vi "IZRCSM_Check_chosen_field (SubVI).vi"(8 "Error In":errorcluster, 11 "Settings in":T2) -> (0 "Error Out":errorcluster, 3 "Settings out":T2)   [LabVIEW 2018]
uses:
  IZRCSM.ctl
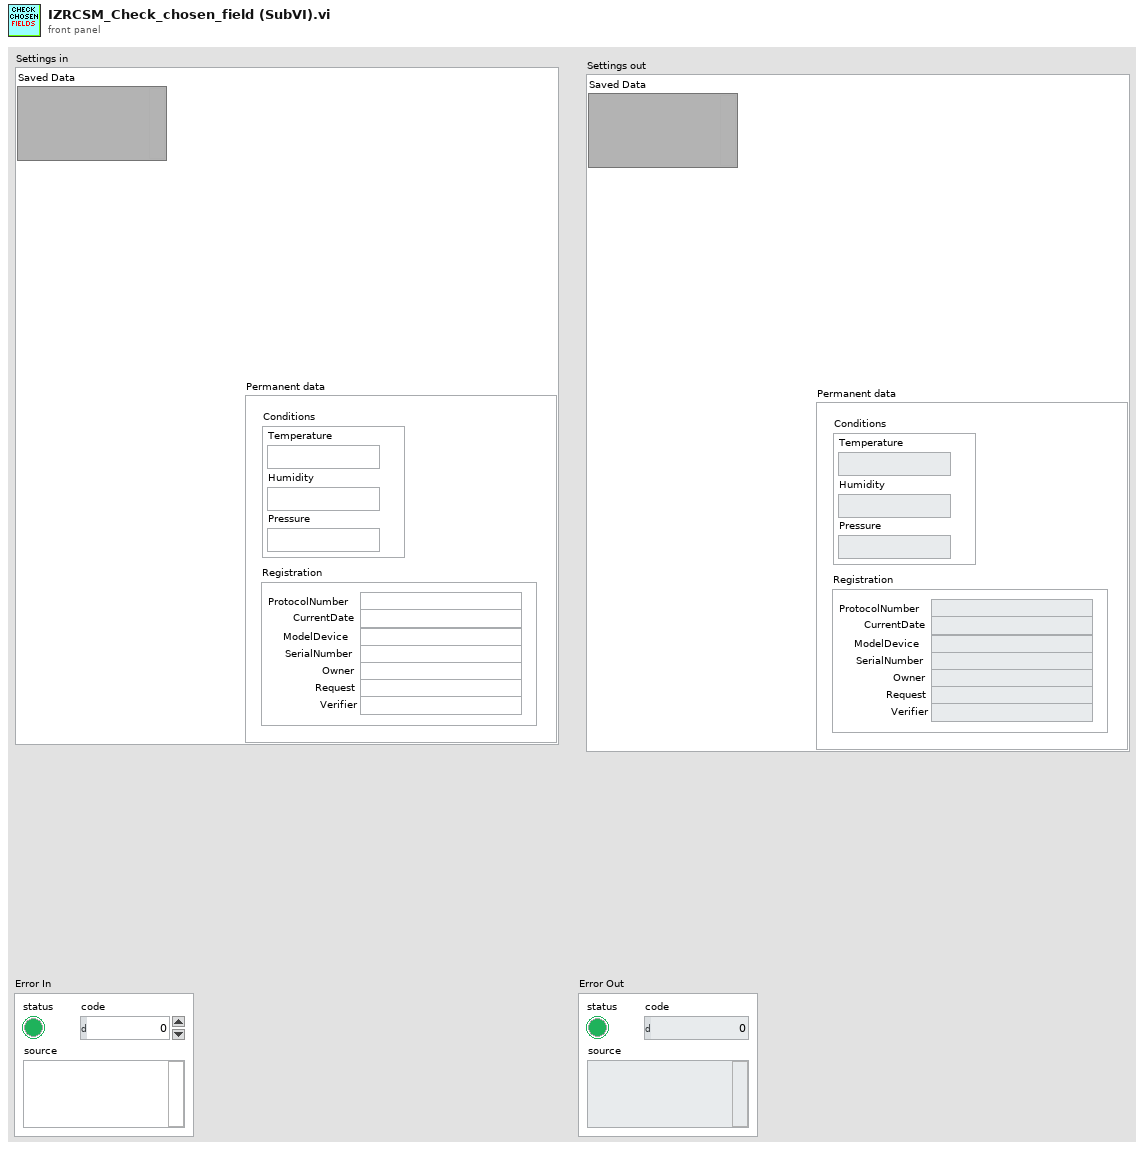
[diagram p1: front panel]
types:
  T1 = typedef "IZRCSM.ctl" = cluster{"Conditions":cluster{"Temperature":string, "Humidity":string, "Pressure":string}, "Registration":cluster{"ProtocolNumber":string, "CurrentDate":string, "ModelDevice":string, "SerialNumber":string, "Owner":string, "Request":string, "Verifier":string}}
  T2 = cluster{"Saved Data":variant, "Permanent data":T1}
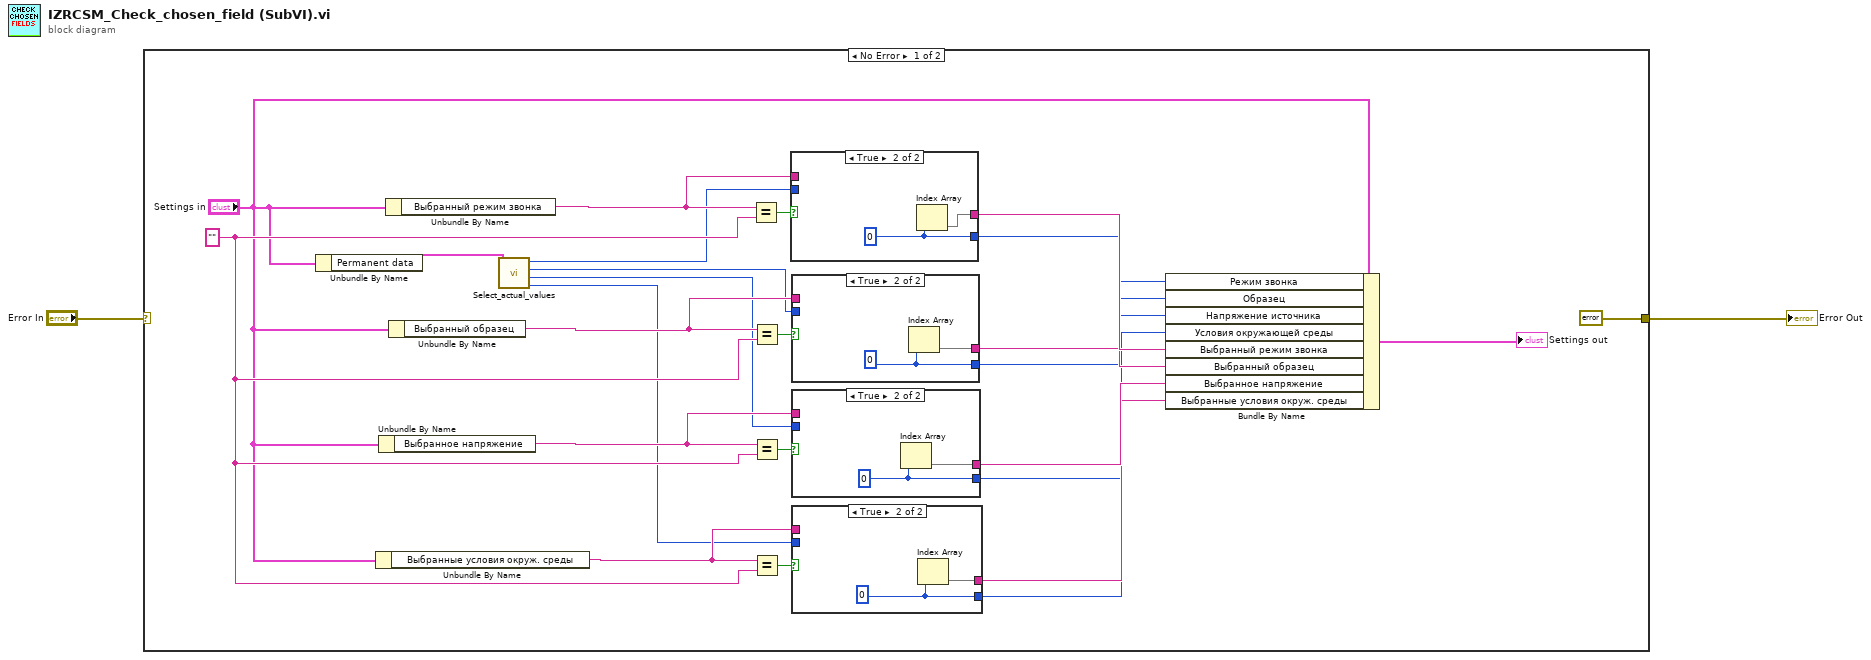
[diagram p0: block diagram]
diagram:
  n1 = case shown="No Error" "Error In" {
    selector: "Error In" -> [_ w48]
    tunnel: [errorcluster {"status"=FALSE, "code"=0, "source"=""} ("error IO") w48] -> w1
    frame No Error {
      w19 = "" ("replace string (\"\")")
      n2 = Unbundle By Name("Settings in") -> ("Permanent data"=w7:T1)
      n3 = Unbundle By Name("Settings in") -> ("Выбранные условия окруж. среды"=w21:string)
      n4 = Unbundle By Name("Settings in") -> ("Выбранное напряжение"=w22:string)
      n5 = Unbundle By Name("Settings in") -> ("Выбранный режим звонка"=w23:string)
      n6 = Unbundle By Name("Settings in") -> ("Выбранный образец"=w24:string)
      n7 = call "Select_actual_values.vi"("CSMinfo in"=w7) -> ("Условия окружающей среды"=w3:u16, "Напряжение источника"=w4:u16, "Образец"=w5:u16, "Режим звонка"=w6:u16)  [unwired: 7 in]
      n8 = Equal?(x=w23, y=w19) -> (x = y?=w27:bool)
      n9 = Equal?(x=w24, y=w19) -> (x = y?=w26:bool)
      n10 = Equal?(x=w22, y=w19) -> (x = y?=w25:bool)
      n11 = Equal?(x=w21, y=w19) -> (x = y?=w20:bool)
      n12 = case shown="True" w27 {
        tunnel: [w44 w46] -> w18
        tunnel: w23 -> [w44 _]
        tunnel: [w43 w45] -> w9
        tunnel: w6 -> [w43 _]
        frame False {
        }
        frame True {
          w45 = 0 ("index")
          n13 = Index Array(index=w45) -> (array=w47:string[], element=w46)
        }
      }
      n14 = case shown="True" w26 {
        tunnel: [w39 w41] -> w17
        tunnel: w24 -> [w39 _]
        tunnel: [w38 w40] -> w10
        tunnel: w5 -> [w38 _]
        frame False {
        }
        frame True {
          w40 = 0 ("index")
          n15 = Index Array(index=w40) -> (array=w42:string[], element=w41)
        }
      }
      n16 = case shown="True" w25 {
        tunnel: [w34 w36] -> w16
        tunnel: w22 -> [w34 _]
        tunnel: [w33 w35] -> w11
        tunnel: w4 -> [w33 _]
        frame False {
        }
        frame True {
          w35 = 0 ("index")
          n17 = Index Array(index=w35) -> (array=w37:string[], element=w36)
        }
      }
      n18 = case shown="True" w20 {
        tunnel: [w29 w31] -> w15
        tunnel: w21 -> [w29 _]
        tunnel: [w28 w30] -> w12
        tunnel: w3 -> [w28 _]
        frame False {
        }
        frame True {
          w30 = 0 ("index")
          n19 = Index Array(index=w30) -> (array=w32:string[], element=w31)
        }
      }
      n20 = Bundle By Name(cluster="Settings in", "Режим звонка"=w9, "Образец"=w10, "Напряжение источника"=w11, "Условия окружающей среды"=w12, "Выбранный режим звонка"=w18, "Выбранный образец"=w17, "Выбранное напряжение"=w16, "Выбранные условия окруж. среды"=w15) -> (→"Settings out":T2)
    }
    frame Error {
    }
  }
  "Error Out" <- w1
